vi "peaks.vi"(8 "error in":errorcluster, 9 "List Parameter Fit in":dbl[][](array[numeric]), 10 "List ROI in":dbl[][](array[numeric]), 11 "Spectrum In":cluster{"Locations":dbl[], "Amplitudes":dbl[]}[](array[cluster])=[{"Locations"=array[8192 elements], "Amplitudes"=array[8192 elements]}, {"Locations"=[0.7467606671708176, 1.9235641208245904, 2.29844815204634, 2.952058877083534, 3.30159027268929, 3.693510427204611, 4.0114062030881295, 5.465964569482503, 5.90533601872882, 6.405158056693529, 7.048430896937822, 7.965886489214608, 8.618241797175692, 9.551852093117594, 10.52313535167255, 11.040953037461485, 11.06991514504198, 11.223209663036432, 12.573413841890297, 13.028543500140618, 13.063940211907648, 13.079189646232502, 13.092703597511122, 13.151136366155567, 13.270484104491407, 13.336875706360313, 14.056987568841034, 14.657535881569391, 15.704563469510273, 16.589800479761752, 17.294355204547227, 18.547875406033366, 19.386017685106246, 23.796403305697343, 24.246601838900926, 24.938407230371723], "Amplitudes"=[8249.877716133802, 11327.172305519029, 56622.259938185096, 7573.210585087449, 5296.252862567521, 568942.2217447343, 85362.57126615923, 5991.635098339018, 7019.466820603001, 22054.8389595985, 7981.806397770608, 3443.0618845857953, 7232.474442522111, 1041.175508376075, 20253.913652049327, 2798.643385245958, 2822.1764574507447, 2760.065665975324, 27847.958569595598, 7072.034132274657, 7057.281156133169, 7080.033735934979, 7084.174530276932, 7080.4596184742295, 7256.269557996548, 7151.769553474873, 10957.376602343933, 8796.257531749367, 4885.946335626738, 151185.40382805822, 73397.38735258923, 16617.278737895518, 11305.024780412065, 1494.0162050533122, 1876.7337579234295, 12601.308465489856]}]) -> (0 "error out":errorcluster, 1 "List ROI out":dbl[][](array[numeric]), 2 "Table":string[][](table), 3 "Peaks Out":cluster{"Locations":dbl[], "Amplitudes":dbl[]}, 4 "List Parameter Fit Out":dbl[][](array[numeric]), 6 "Spectrum Fitted":cluster{"Array":dbl[], "Array":dbl[]})   [LabVIEW 2023]
uses:
  <vilib>/Utility/miscctls.llb/LVCursorListTypeDef.ctl
  <vilib>/Utility/miscctls.llb/LVPoint32TypeDef.ctl
  control/global name path.vi
  <vilib>/Utility/cursorutil.llb/Set Cursor (Icon Pict).vi
  <vilib>/Utility/file.llb/Write Delimited Spreadsheet (DBL).vi
  <vilib>/Utility/file.llb/Write Delimited Spreadsheet (string).vi
  <vilib>/Utility/file.llb/Read Delimited Spreadsheet (string).vi
  <vilib>/Utility/file.llb/Read Delimited Spreadsheet (DBL).vi
  queue/Front Panel Message Queue.lvlib
panel:
  out "ROIs":string[][](table)
  out "reference fit panel":refnum<vi>
  in  "previous cursor ID":refnum<k1>
  in  "open":bool
  in  "save":bool
  in  "reset":bool
  out "cluster roi":T1
  in  "mapping":enum16{"Y -Linear", "Y - Log"}(ring)
  in  "eval":bool
  out "grabbing":bool
  in  "Delete":bool
  in  "Normal":bool
  in  "fit":bool
  out "removing":bool
  in  "Stop":bool
  out "Spectrum":cluster{"Locations":dbl[], "Amplitudes":dbl[]}[](graph)
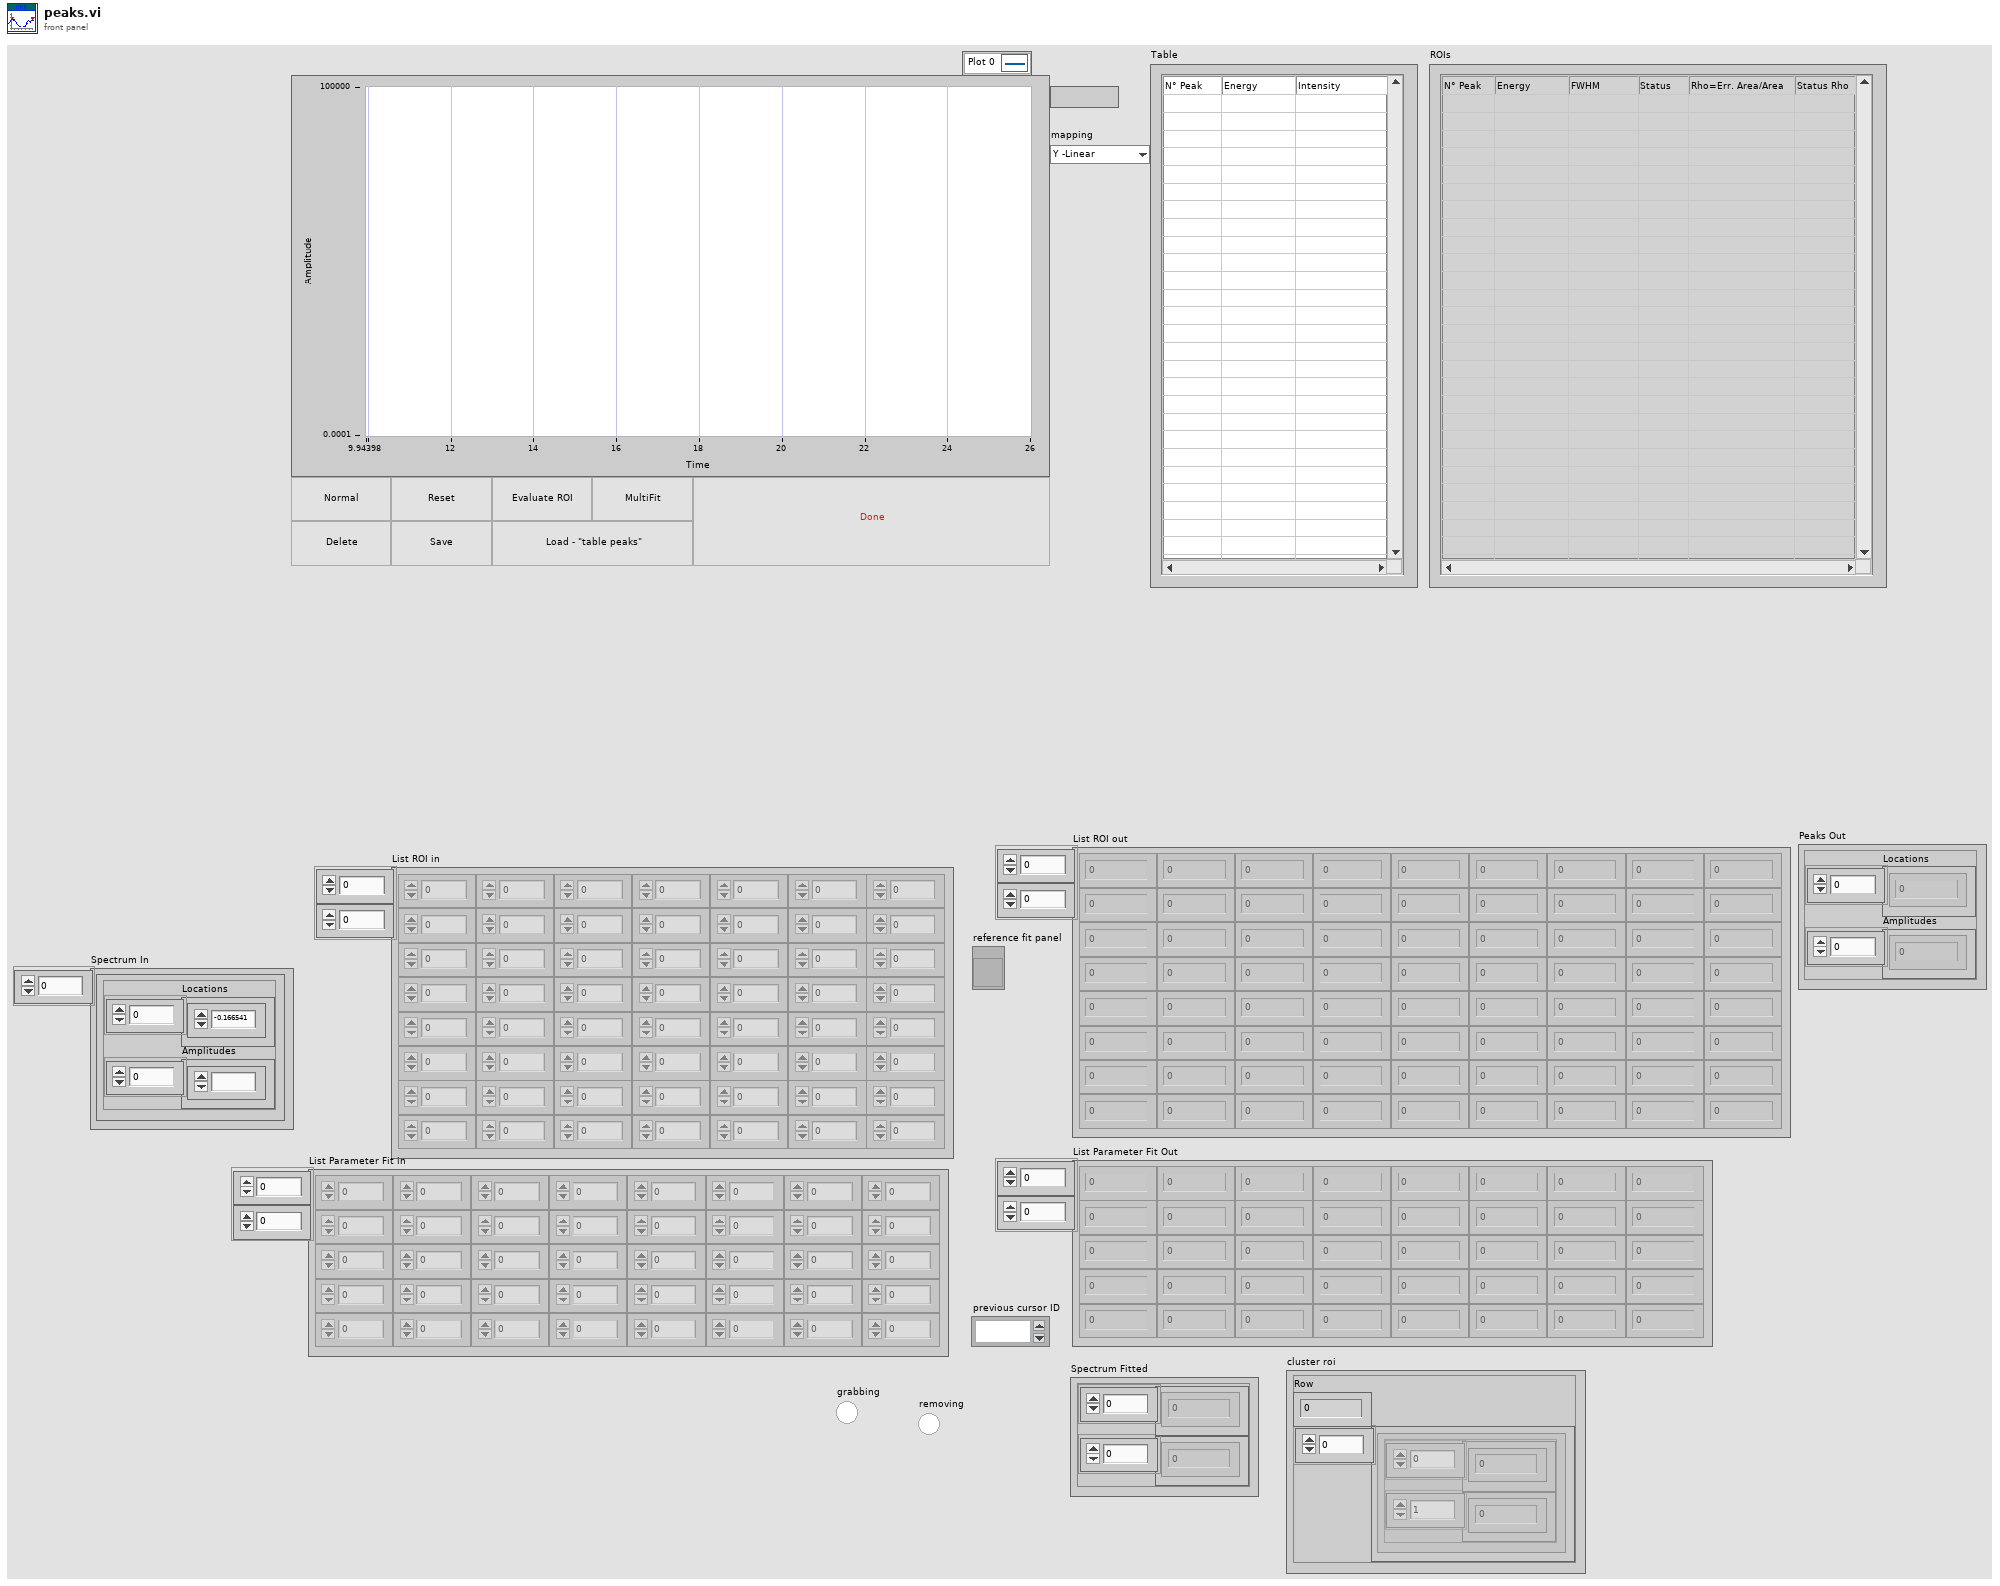
[diagram p1: front panel]
types:
  T1 = cluster{"Row":i32, "Array":cluster{"Array":dbl[], "Array":dbl[]}[]}
  T2 = typedef "Front Panel Message Queue.lvlib/load Message Queues.ctl" = cluster{"Main":refnum<queue>}
  T3 = enum32{"Invalid", "Standard", "Closed", "Hidden", "Minimized", "Maximized"}
  T4 = cluster{"Name":string, "Color":u32, "Style":i32, "Point Style":i32, "Name Visible":bool, "Allow Drag":bool, "Cursor Mode":u32, "Plot":i32, "Index":i32, "Position":cluster{"X":dbl, "Y":dbl}, "X Scale":u32, "Y Scale":u32, "Watch Plots":i32[], "Watch All Plots":bool, "Plot Area":i32, "Label Offset":cluster{"X":dbl, "Y":dbl}}
  T5 = typedef "LVCursorListTypeDef.ctl" = cluster{"Name":string, "Color":u32, "Style":u8, "Point Style":u8, "Name Visible":bool, "Allow Drag":bool, "Cursor Mode":u32, "Plot":i32, "Index":i32, "Position":cluster{"X":dbl, "Y":dbl}, "X Scale":u32, "Y Scale":u32, "Watch Plots":i32[], "Watch All Plots":bool, "Plot Area":i32, "Label Offset":cluster{"X":dbl, "Y":dbl}}[]
  T6 = typedef "LVPoint32TypeDef.ctl" = cluster{"Horizontal":i32, "Vertical":i32}
  T7 = cluster{"Name":string, "Color":u32, "Style":i32, "Point Style":i32, "Name Visible":bool, "Allow Drag":bool, "Cursor Mode":u32, "Plot":i32, "Index":i32, "Position":cluster{"X":dbl, "Y":dbl}, "X Scale":u32, "Y Scale":u32, "Watch Plots":i32[], "Watch All Plots":bool, "Plot Area":i32, "Label Offset":cluster{"X":dbl, "Y":dbl}}[]
  T8 = typedef "LVRowAndColumnTypeDef.ctl" = cluster{"Row":i32, "Column":i32}
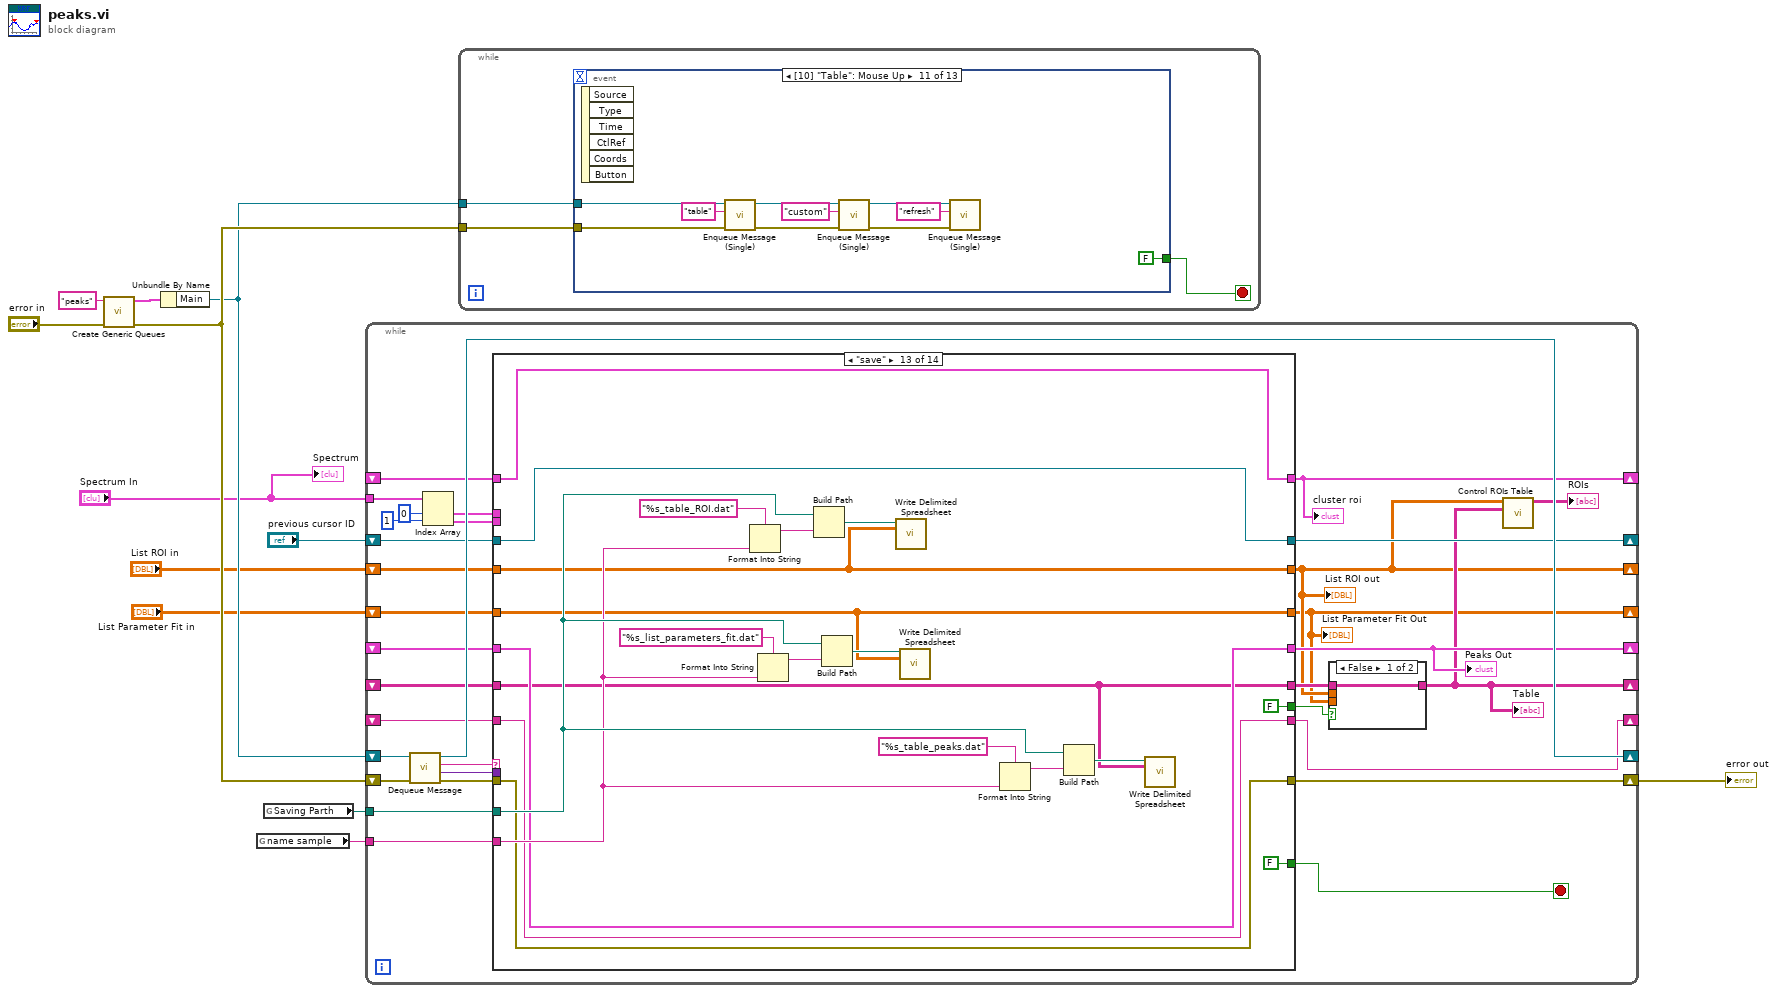
[diagram p0: block diagram]
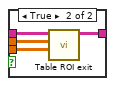
[diagram p2: hidden frame]
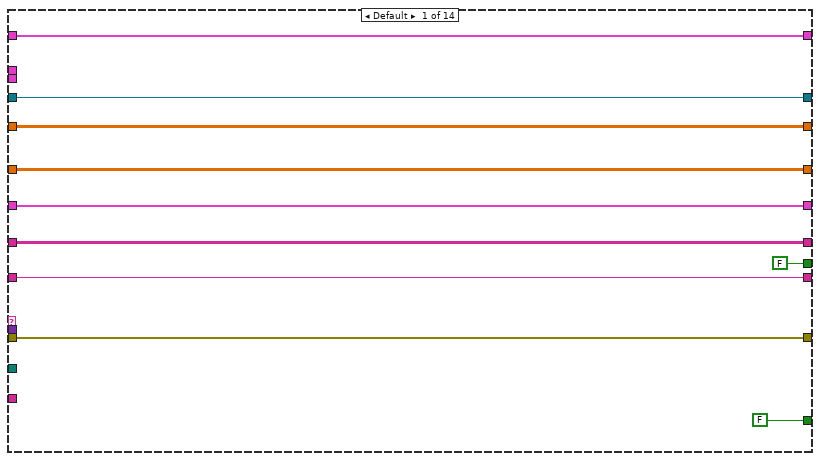
[diagram p3: hidden frame]
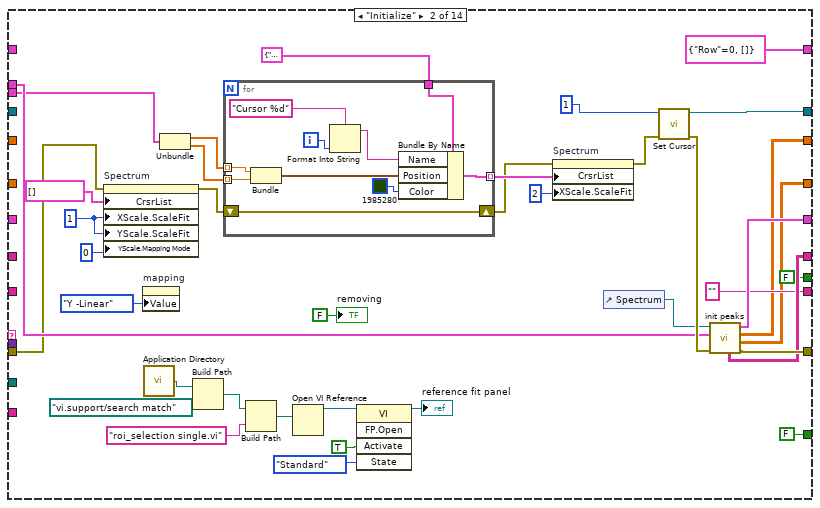
[diagram p4: hidden frame]
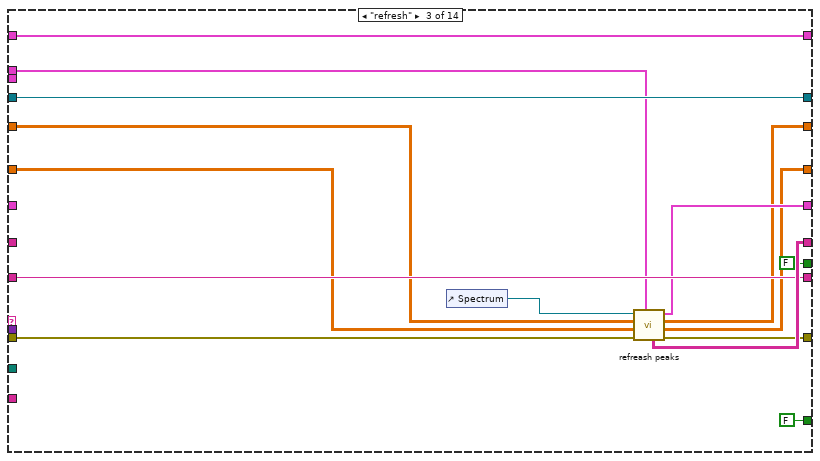
[diagram p5: hidden frame]
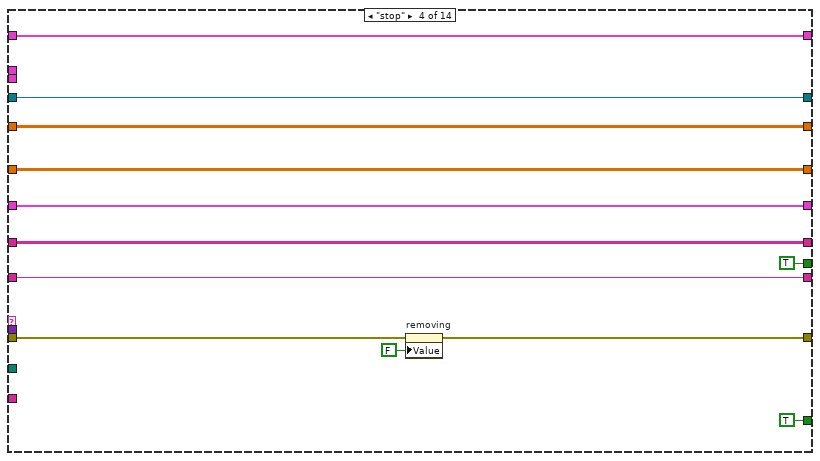
[diagram p6: hidden frame]
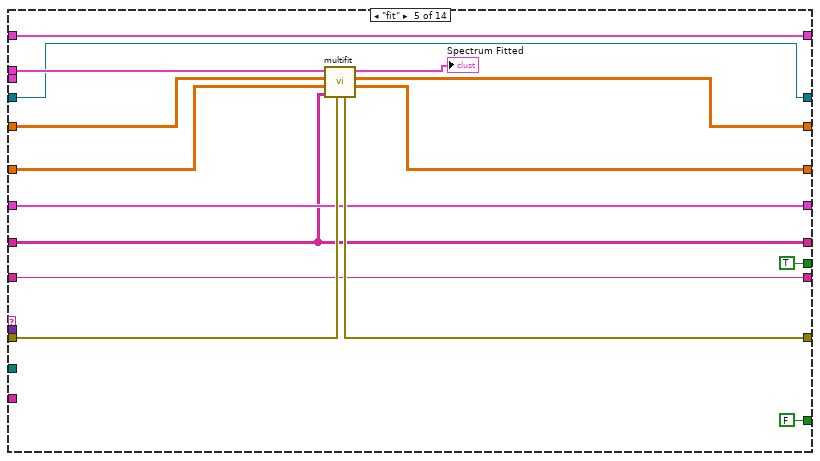
[diagram p7: hidden frame]
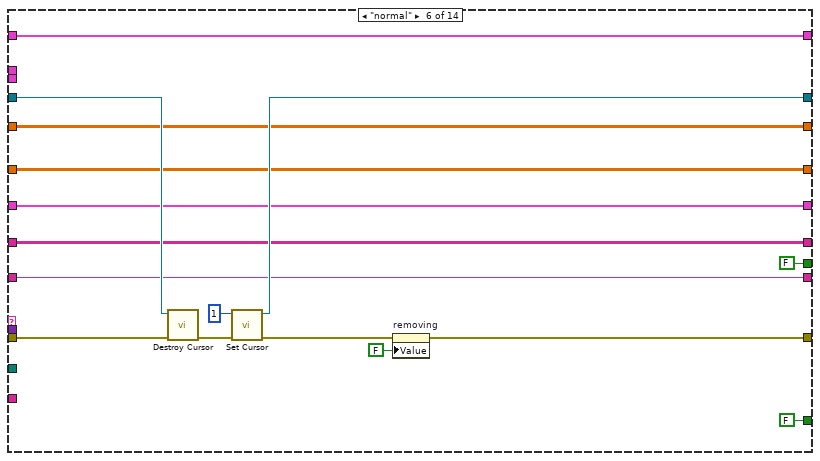
[diagram p8: hidden frame]
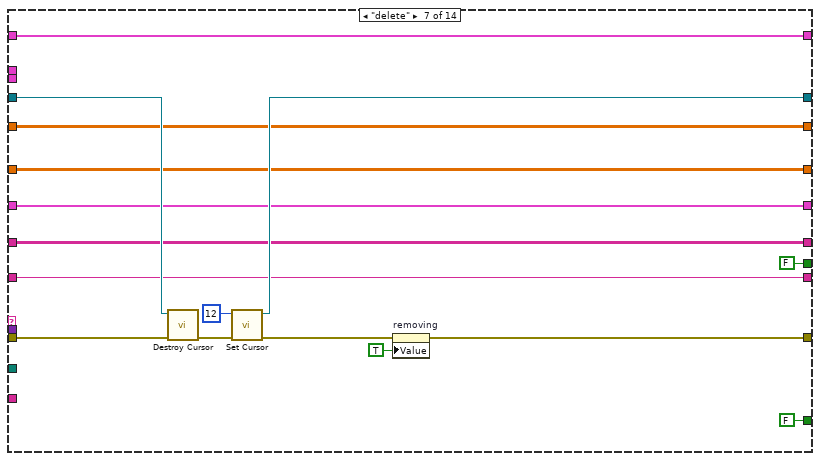
[diagram p9: hidden frame]
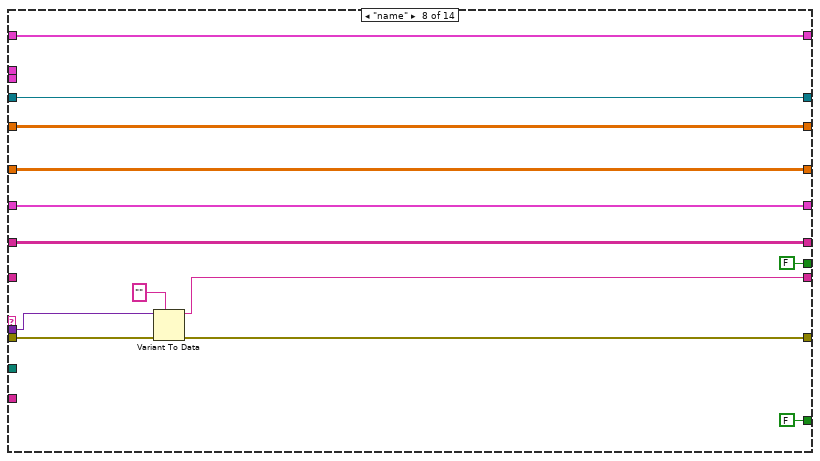
[diagram p10: hidden frame]
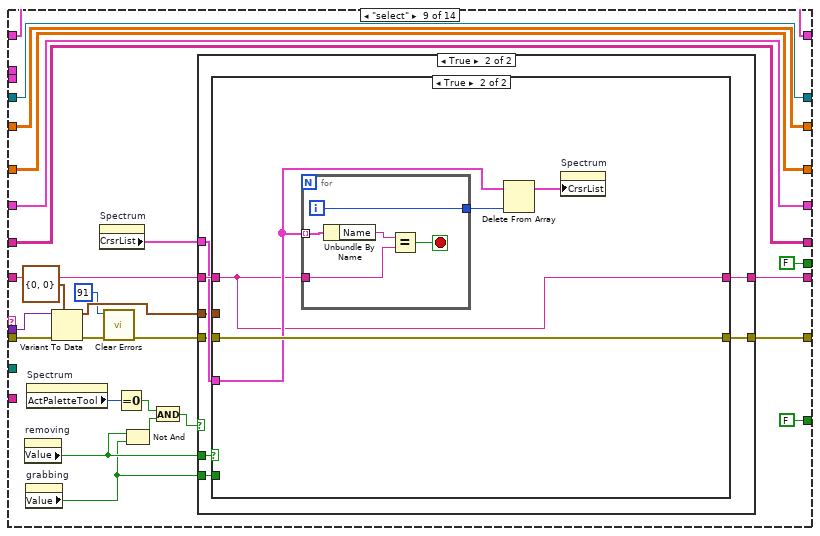
[diagram p11: hidden frame]
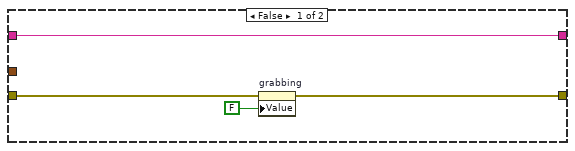
[diagram p12: hidden frame]
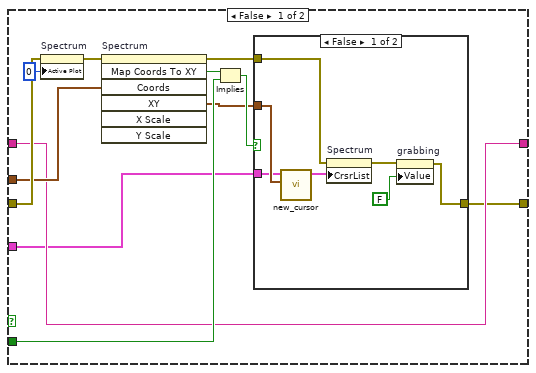
[diagram p13: hidden frame]
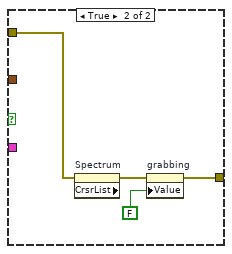
[diagram p14: hidden frame]
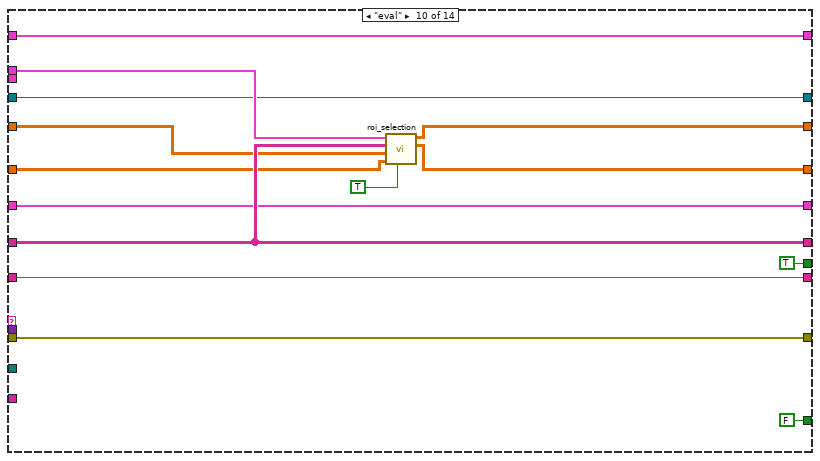
[diagram p15: hidden frame]
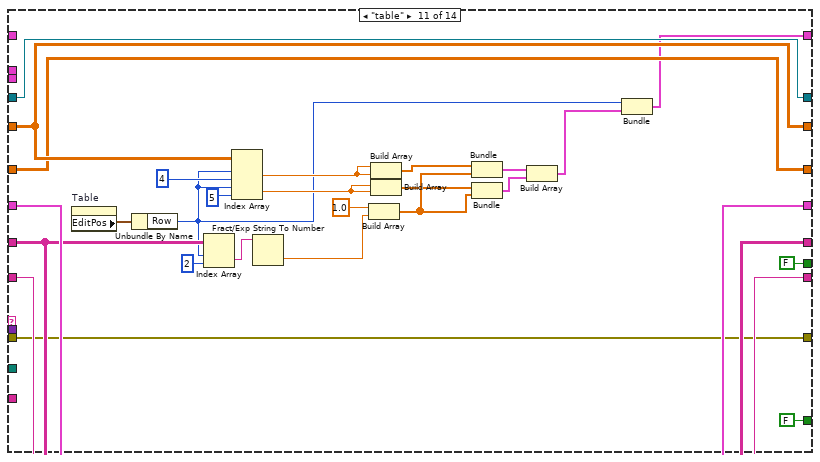
[diagram p16: hidden frame]
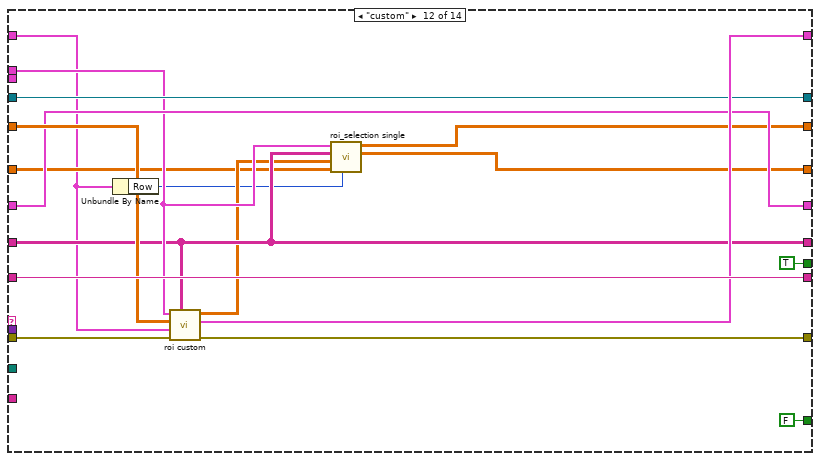
[diagram p17: hidden frame]
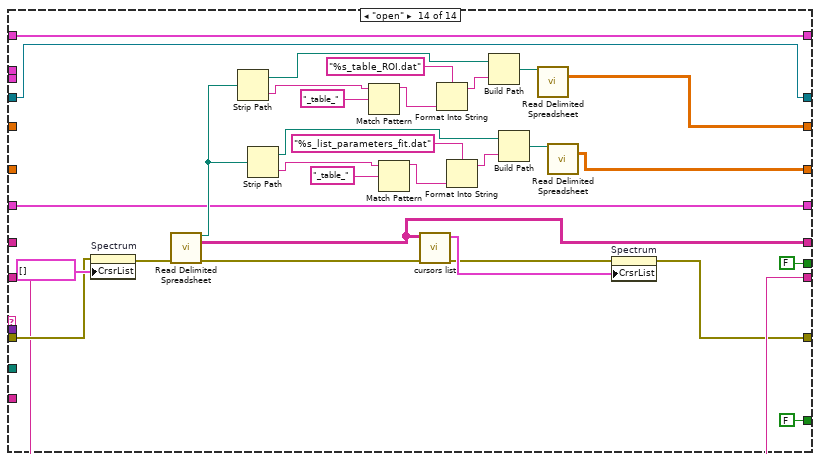
[diagram p18: hidden frame]
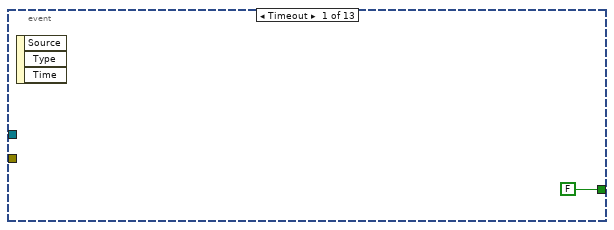
[diagram p19: hidden frame]
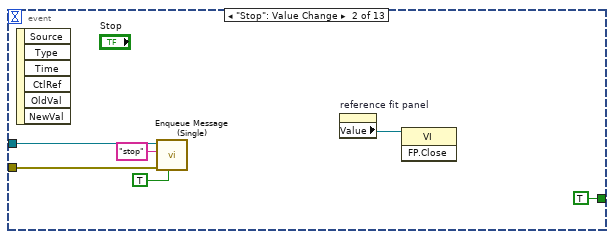
[diagram p20: hidden frame]
diagram:
  n1 = call "Create Generic Queues.vi"("error in (no error)"="error in", "name"="peaks") -> ("error out"=w10:errorcluster, "Message Queues"=w9:T2)  [unwired: 8 in]
  n2 = Unbundle By Name(w9) -> ("Main"=w8:refnum<queue>)
  n3 = global read "global name path.vi" "name sample"() -> (w4:string)
  n4 = global read "global name path.vi" "Saving Parth"() -> (w5:path)
  n5 = while {
    shift-right: [w42] -> _
    shift-left: w8 -> [w43]
    shift-right: [w39] -> w6
    shift-left: w10 -> [w44]
    tunnel: "Spectrum In" -> [w28]
    tunnel: w5 -> [w35]
    tunnel: w4 -> [w36]
    shift-right: [w34] -> _
    shift-left: "previous cursor ID" -> [w33]
    shift-right: [w16] -> _
    shift-left: "List ROI in" -> [w30]
    shift-right: [w15] -> _
    shift-left: "List Parameter Fit in" -> [w29]
    shift-right: [w20] -> _
    shift-left: _ -> [w32]
    shift-right: [w18] -> _
    shift-left: _ -> [w31]
    shift-right: [w14] -> _
    shift-left: _ -> [w23]
    shift-right: [w21] -> _
    shift-left: _ -> [w22]
    stop <- w38 stop-if-true
    n6 = call "Dequeue Message.vi"("error in (no error)"=w44, "Message Queue"=w43) -> ("error out"=w40:errorcluster, "Message Data"=w37:variant, "Message"=w41:string, "dup Message Queue"=w42:refnum<queue>)  [unwired: 5 in, 1 out]
    n7 = Index Array(array=w28, index #1=0 ("index"), index #2=1 ("index")) -> (element #1=w25:cluster{"Locations":dbl[], "Amplitudes":dbl[]}, element #2=w24:cluster{"Locations":dbl[], "Amplitudes":dbl[]})
    n8 = case shown="\"save\"" w41 {
      tunnel: w40 -> [w59 w75 w119 w129 w145 w162 w178 w193 w218 w272 w285 w320 w330 w371]
      tunnel: [w59 w85 w113 w130 w144 w154 w170 w189 w215 w272 w285 w319 w330 w344] -> w39
      tunnel: [FALSE FALSE FALSE TRUE FALSE FALSE FALSE FALSE FALSE FALSE FALSE FALSE FALSE FALSE] -> w38
      tunnel: w37 -> [_ _ _ _ _ _ _ w192 w217 _ _ _ _ _]
      tunnel: w36 -> [_ _ _ _ _ _ _ _ _ _ _ _ w332 _]
      tunnel: w35 -> [_ _ _ _ _ _ _ _ _ _ _ _ w333 _]
      tunnel: [w57 w86 w121 w133 w147 w160 w176 w184 w212 w268 w301 w314 w326 w349] -> w34
      tunnel: w33 -> [w57 _ w121 w133 w147 w161 w177 w184 w212 w268 w301 w314 w326 w349]
      tunnel: [w56 w74 w115 w125 w137 w159 w175 w185 w211 w269 w294 w306 w324 w353] -> w16
      tunnel: [w55 w73 w114 w124 w138 w158 w174 w186 w210 w270 w293 w307 w323 w352] -> w15
      tunnel: [w54 w82 w116 w132 w142 w157 w173 w187 w209 w267 w302 w315 w328 w351] -> w20
      tunnel: w32 -> [w54 _ _ w132 w142 w157 w173 w187 w209 w267 w302 w315 w328 w351]
      tunnel: [w53 w81 w118 w126 w136 w156 w172 w188 w208 w276 w297 w312 w325 w347] -> w17
      tunnel: w31 -> [w53 _ _ w126 w136 w156 w172 w188 w208 w276 w297 w312 w325 _]
      tunnel: w30 -> [w56 _ w110 w125 w148 w159 w175 w185 w211 w275 w294 w317 w324 _]
      tunnel: w29 -> [w55 _ w109 w124 w143 w158 w174 w186 w210 w274 w293 w310 w323 _]
      tunnel: w25 -> [_ w79 w111 _ w149 _ _ _ _ w277 _ w313 _ _]
      tunnel: w24 -> [_ w78 _ _ _ _ _ _ _ _ _ _ _ _]
      tunnel: [w52 "" w117 w128 w140 w152 w168 w190 w206 w271 w303 w318 w329 w370] -> w14
      tunnel: w23 -> [w52 _ w117 w128 w140 w152 w168 _ w207 w271 w303 w318 w329 w370]
      tunnel: [w51 cluster{"Row":i32, cluster{dbl[], dbl[]}[]} {"Row"=0, []} w112 w127 w139 w151 w167 w183 w205 w266 w280 w316 w327 w350] -> w21
      tunnel: w22 -> [w51 _ w112 w127 w139 w151 w167 w183 w205 w266 _ w309 w327 w350]
      tunnel: [FALSE FALSE FALSE TRUE TRUE FALSE FALSE FALSE FALSE TRUE FALSE TRUE FALSE FALSE] -> w13
      frame Default {
      }
      frame "Initialize" {
        w96 = u8 1 ("X Scale.Scale Fit")
        n9 = property on="Spectrum" class="XYGraph (strict)"(error in=w75, "CrsrList"=T5 [] ("Cursor List"), "XScale.ScaleFit"=w96, "YScale.ScaleFit"=w96, "YScale.Mapping Mode"=u8 0 ("Y Scale.Mapping Mode")) -> (error out=w91:errorcluster)  [unwired: 1 in, 1 out]
        n10 = property on="mapping" class="Enum (strict)"("Value"=enum16{"Y -Linear", "Y - Log"}."Y -Linear" ("mapping")) -> ()  [unwired: 2 in, 2 out]
        n11 = call <vilib>:"Application Directory.vi"() -> ("Application Directory"=w70:path)
        n12 = Unbundle(w78) -> ("Locations"=w93:dbl[], "Amplitudes"=w92:dbl[])
        n13 = Build Path(base path=w70, name or relative path=path "vi.support/search match") -> (appended path=w67:path)
        n14 = for {
          tunnel: w93 -> [w105] mode=indexing
          tunnel: w92 -> [w104] mode=indexing
          tunnel: T4 {"Name"="", "Color"=16776704, "Style"=4, "Point Style"=13, "Name Visible"=FALSE, "Allow Drag"=TRUE, "Cursor Mode"=0, "Plot"=0, "Index"=0, "Position"={"X"=0.0, "Y"=0.0}, "X Scale"=0, "Y Scale"=0, "Watch Plots"=[], "Watch All Plots"=FALSE, "Plot Area"=0, "Label Offset"={"X"=0.0, "Y"=0.0}} -> [w103]
          tunnel: [w99] -> w90 mode=indexing
          shift-right: [w98] -> w89
          shift-left: w91 -> [w98]
          i -> [w106]
          n15 = Bundle("Numeric Control"=w105, "Numeric"=w104) -> (w100:cluster{"Numeric Control":dbl, "Numeric":dbl})  [unwired: 1 in]
          n16 = Format Into String(format string="Cursor %d", w106) -> (resulting string=w102:string)  [unwired: 2 in, 1 out]
          n17 = Bundle By Name(cluster=w103, "Name"=w102, "Position"=w100, "Color"=u32 1985280) -> (w99:T4)
        }
        n18 = Build Path(base path=w67, name or relative path="roi_selection single.vi") -> (appended path=w66:path)
        n19 = Open VI Reference(vi path=w66) -> (vi reference=w65:refnum<vi>)  [unwired: 5 in, 1 out]
        n20 = invoke class="VI" method="FP.Open"(reference=w65, "Activate"=TRUE ("Activate?"), "State"=T3."Standard") -> (reference out=→"reference fit panel":refnum<vi>)  [unwired: 2 in, 4 out]
        n21 = property on="Spectrum" class="XYGraph (strict)"(error in=w89, "CrsrList"=w90, "XScale.ScaleFit"=u8 2 ("X Scale.Scale Fit")) -> (error out=w88:errorcluster)  [unwired: 1 in, 1 out]
        n22 = control-ref of="Spectrum"() -> (w83:refnum<vi>)
        n23 = call-poly <vilib>:"Set Cursor.vi"("error in (no error)"=w88, "icon"=u16 1) -> ("error out"=w84:errorcluster, "previous cursor ID"=w86:refnum<k1>)  [unwired: 8 in]
        n24 = call "init peaks.vi"("error in"=w84, "element"=w79, "Spectrum"=w83) -> ("error out"=w85:errorcluster, "List Parameter Fit Out"=w73:dbl[][], "List ROI Out"=w74:dbl[][], "Peaks Out"=w82:cluster{"Locations":dbl[], "Amplitudes":dbl[]}, "Table"=w81:string[][])  [unwired: 4 in]
        "removing" <- FALSE ("removing")
      }
      frame "refresh" {
        n25 = control-ref of="Spectrum"() -> (w120:refnum<vi>)
        n26 = call "refreash peaks.vi"("element"=w111, "error in"=w119, "List Parameter Fit in"=w109, "List ROI in"=w110, "Spectrum"=w120) -> ("error out"=w113:errorcluster, "List Parameter Fit Out"=w114:dbl[][], "List ROI Out"=w115:dbl[][], "Peaks Out"=w116:cluster{"Locations":dbl[], "Amplitudes":dbl[]}, "Table"=w118:string[][])  [unwired: 2 in]
      }
      frame "stop" {
        n27 = property on="removing" class="Bool (strict)"(error in=w129, "Value"=FALSE ("removing")) -> (error out=w130:errorcluster)  [unwired: 1 in, 1 out]
      }
      frame "fit" {
        n28 = call "multifit.vi"("error in"=w145, "List Peaks"=w136, "List Parameter Fit In"=w143, "List ROI In"=w148, "Spectrum In"=w149) -> ("List Parameter Fit Out"=w138:dbl[][], "List ROI Out"=w137:dbl[][], "Spectrum Fitted"=→"Spectrum Fitted":cluster{"Array":dbl[], "Array":dbl[]}, "error out"=w144:errorcluster)  [unwired: 3 in]
      }
      frame "normal" {
        n29 = call <vilib>:"Destroy Cursor.vi"("cursor ID"=w161, "error in (no error)"=w162) -> ("error out"=w163:errorcluster)  [unwired: 8 in]
        n30 = call-poly <vilib>:"Set Cursor.vi"("error in (no error)"=w163, "icon"=u16 1 ("Cursor Icon")) -> ("error out"=w153:errorcluster, "previous cursor ID"=w160:refnum<k1>)  [unwired: 8 in]
        n31 = property on="removing" class="Bool (strict)"(error in=w153, "Value"=FALSE ("removing")) -> (error out=w154:errorcluster)  [unwired: 1 in, 1 out]
      }
      frame "delete" {
        n32 = call <vilib>:"Destroy Cursor.vi"("cursor ID"=w177, "error in (no error)"=w178) -> ("error out"=w179:errorcluster)  [unwired: 8 in]
        n33 = call-poly <vilib>:"Set Cursor.vi"("error in (no error)"=w179, "icon"=u16 12 ("Cursor Icon")) -> ("error out"=w169:errorcluster, "previous cursor ID"=w176:refnum<k1>)  [unwired: 8 in]
        n34 = property on="removing" class="Bool (strict)"(error in=w169, "Value"=TRUE ("removing")) -> (error out=w170:errorcluster)  [unwired: 1 in, 1 out]
      }
      frame "name" {
        n35 = Variant To Data(error in=w193, type="", Variant=w192) -> (data=w190:string, error out=w189:errorcluster)
      }
      frame "select" {
        n36 = property on="removing" class="Bool (strict)"() -> ("Value"=w200:bool)  [unwired: 2 in, 2 out]
        n37 = property on="grabbing" class="Bool (strict)"() -> ("Value"=w199:bool)  [unwired: 2 in, 2 out]
        n38 = property on="Spectrum" class="XYGraph (strict)"() -> ("ActPaletteTool"=w216:i32)  [unwired: 2 in, 2 out]
        n39 = Variant To Data(error in=w218, type=T6 {"Horizontal"=0, "Vertical"=0} ("Coords"), Variant=w217) -> (data=w214:T6, error out=w203:errorcluster)
        n40 = property on="Spectrum" class="XYGraph (strict)"() -> ("CrsrList"=w213:T5)  [unwired: 2 in, 2 out]
        n41 = call <vilib>:"Clear Errors.vi"("error in (no error)"=w203, "specific error code to clear (0: all)"=91) -> ("error out"=w202:errorcluster)  [unwired: 4 in, 1 out]
        n42 = Equal To 0?(x=w216) -> (x = 0?=w198:bool)
        n43 = Not And(1:w199, 2:w200) -> (0:w197:bool)
        n44 = And(x=w198, y=w197) -> (x .and. y?=w196:bool)
        n45 = case shown="True" w196 {
          tunnel: w202 -> [w221 w227]
          tunnel: [w220 w228] -> w215
          tunnel: w214 -> [_ w225]
          tunnel: w213 -> [_ w229]
          tunnel: w207 -> [w223 w230]
          tunnel: w200 -> [_ w231]
          tunnel: [w223 w226] -> w206
          tunnel: w199 -> [_ w224]
          frame False {
            n46 = property on="grabbing" class="Bool (strict)"(error in=w221, "Value"=FALSE ("grabbing")) -> (error out=w220:errorcluster)  [unwired: 1 in, 1 out]
          }
          frame True {
            n47 = case shown="True" w231 {
              tunnel: w230 -> [w237 w255]
              tunnel: w229 -> [w233 w257]
              tunnel: [w235 w259] -> w228
              tunnel: w227 -> [w242 w259]
              tunnel: [w237 w255] -> w226
              tunnel: w225 -> [w240 _]
              tunnel: w224 -> [w238 _]
              frame False {
                n48 = property on="Spectrum" class="XYGraph (strict)"(error in=w242, "Active Plot"=u32 0) -> (error out=w241:errorcluster)  [unwired: 1 in, 1 out]
                n49 = invoke on="Spectrum" class="XYGraph (strict)" method="Map Coords To XY"(error in=w241, "Coords"=w240) -> (error out=w234:errorcluster, "Map Coords To XY"=w239:bool, "XY"=w232:cluster{"X":dbl, "Y":dbl})  [unwired: 5 in, 4 out]
                n50 = Implies(1:w238, 2:w239) -> (0:w236:bool)
                n51 = case shown="False" w236 {
                  tunnel: [w244 w251] -> w235
                  tunnel: w234 -> [w247 w254]
                  tunnel: w233 -> [w249 _]
                  tunnel: w232 -> [w250 _]
                  frame False {
                    n52 = call "new_cursor.vi"("XY"=w250, "CrsrList"=w249) -> ("CrsrList Out"=w248:T7)  [unwired: 9 in]
                    n53 = property on="Spectrum" class="XYGraph (strict)"(error in=w247, "CrsrList"=w248) -> (error out=w246:errorcluster)  [unwired: 1 in, 1 out]
                    n54 = property on="grabbing" class="Bool (strict)"(error in=w246, "Value"=FALSE ("grabbing")) -> (error out=w244:errorcluster)  [unwired: 1 in, 1 out]
                  }
                  frame True {
                    n55 = property on="Spectrum" class="XYGraph (strict)" props=["CrsrList"](error in=w254) -> (error out=w252:errorcluster)  [unwired: 1 in, 2 out]
                    n56 = property on="grabbing" class="Bool (strict)"(error in=w252, "Value"=FALSE ("grabbing")) -> (error out=w251:errorcluster)  [unwired: 1 in, 1 out]
                  }
                }
              }
              frame True {
                n57 = for {
                  tunnel: w257 -> [w264] mode=indexing
                  tunnel: w255 -> [w262]
                  tunnel: [w260] -> w258
                  i -> [w260]
                  stop <- w261 stop-if-true
                  n58 = Unbundle By Name(w264) -> ("Name"=w263:string)
                  n59 = Equal?(x=w263, y=w262) -> (x = y?=w261:bool)
                }
                n60 = Delete From Array(array=w257, index=w258) -> (array with subset deleted=w256:T5)  [unwired: 1 in, 1 out]
                n61 = property on="Spectrum" class="XYGraph (strict)"("CrsrList"=w256) -> ()  [unwired: 2 in, 2 out]
              }
            }
          }
        }
      }
      frame "eval" {
        n62 = call "roi_selection.vi"("Starting Evaluate?"=TRUE, "List Parameter Fit In"=w274, "List ROI In"=w275, "List Peaks"=w276, "Spectrum In"=w277) -> ("List Parameter Fit Out"=w270:dbl[][], "List ROI Out"=w269:dbl[][])  [unwired: 5 in]
      }
      frame "table" {
        n63 = property on="Table" class="Tbl (strict)"() -> ("EditPos"=w300:T8)  [unwired: 2 in, 2 out]
        n64 = Unbundle By Name(w300) -> ("Row"=w281:i32)
        n65 = Index Array(array=w297, index (row)=w281, index (col)=2 ("disabled index (col)")) -> (element=w299:string)
        n66 = Index Array(array=w294, index (row) #1=w281, index (col) #1=4 ("disabled index (col)"), index (row) #2=w281, index (col) #2=5 ("disabled index (col)")) -> (element #1=w288:dbl, element #2=w287:dbl)
        n67 = Fract/Exp String To Number(string=w299) -> (number=w286:dbl)  [unwired: 3 in, 1 out]
        n68 = Build Array(1.0, w286) -> (w292:dbl[])
        n69 = Build Array(w288, w288) -> (w289:dbl[])
        n70 = Build Array(w287, w287) -> (w291:dbl[])
        n71 = Bundle(w289, w292) -> (w284:cluster{dbl[], dbl[]})  [unwired: 1 in]
        n72 = Bundle(w291, w292) -> (w283:cluster{dbl[], dbl[]})  [unwired: 1 in]
        n73 = Build Array(w284, w283) -> (w282:cluster{dbl[], dbl[]}[])
        n74 = Bundle("Row"=w281, w282) -> (w280:cluster{"Row":i32, cluster{dbl[], dbl[]}[]})  [unwired: 1 in]
      }
      frame "custom" {
        n75 = Unbundle By Name(w309) -> ("Row"=w308:i32)
        n76 = call "roi custom.vi"("Table"=w312, "Error In"=w320, "Cluster roi in"=w309, "List ROI In"=w317, "Spectrum In"=w313) -> ("Error Out"=w319:errorcluster, "Cluster roi out"=w316:T1, "List ROI Out"=w311:dbl[][])  [unwired: 4 in]
        n77 = call "roi_selection single.vi"("Peak selected"=w308, "List Parameter Fit In"=w310, "List ROI In"=w311, "List Peaks"=w312, "Spectrum In"=w313) -> ("List Parameter Fit Out"=w307:dbl[][], "List ROI Out"=w306:dbl[][])  [unwired: 5 in]
      }
      frame "save" {
        n78 = Format Into String(format string="%s_table_ROI.dat", w332) -> (resulting string=w342:string)  [unwired: 2 in, 1 out]
        n79 = Format Into String(format string="%s_list_parameters_fit.dat", w332) -> (resulting string=w336:string)  [unwired: 2 in, 1 out]
        n80 = Build Path(base path=w333, name or relative path=w342) -> (appended path=w340:path)
        n81 = Build Path(base path=w333, name or relative path=w336) -> (appended path=w334:path)
        n82 = call-poly <vilib>:"Write Delimited Spreadsheet.vi"("file path (dialog if empty)"=w340, "2D data"=w324) -> ()  [unwired: 12 in, 2 out]
        n83 = call-poly <vilib>:"Write Delimited Spreadsheet.vi"("file path (dialog if empty)"=w334, "2D data"=w323) -> ()  [unwired: 12 in, 2 out]
        n84 = Format Into String(format string="%s_table_peaks.dat", w332) -> (resulting string=w337:string)  [unwired: 2 in, 1 out]
        n85 = Build Path(base path=w333, name or relative path=w337) -> (appended path=w339:path)
        n86 = call-poly <vilib>:"Write Delimited Spreadsheet.vi"("file path (dialog if empty)"=w339, "2D data"=w325) -> ()  [unwired: 12 in, 2 out]
      }
      frame "open" {
        n87 = property on="Spectrum" class="XYGraph (strict)"(error in=w371, "CrsrList"=T5 [] ("Cursor List")) -> (error out=w372:errorcluster)  [unwired: 1 in, 1 out]
        n88 = call-poly <vilib>:"Read Delimited Spreadsheet.vi"("error in (no error)"=w372) -> ("new file path (Not A Path if cancelled)"=w354:path, "all rows"=w347:string[][], "error out"=w348:errorcluster)  [unwired: 9 in, 3 out]
        n89 = Strip Path(path=w354) -> (stripped path=w367:path, name=w365:string)
        n90 = Strip Path(path=w354) -> (stripped path=w356:path, name=w358:string)
        n91 = Match Pattern(string=w365, regular expression="_table_" ("format string")) -> (before substring=w364:string)  [unwired: 1 in, 3 out]
        n92 = Match Pattern(string=w358, regular expression="_table_" ("format string")) -> (before substring=w359:string)  [unwired: 1 in, 3 out]
        n93 = call "cursors list.vi"("error in"=w348, "Table"=w347) -> ("error out"=w345:errorcluster, "Cursors List"=w346:T7)  [unwired: 8 in]
        n94 = Format Into String(format string="%s_table_ROI.dat", w364) -> (resulting string=w366:string)  [unwired: 2 in, 1 out]
        n95 = Format Into String(format string="%s_list_parameters_fit.dat", w359) -> (resulting string=w357:string)  [unwired: 2 in, 1 out]
        n96 = Build Path(base path=w367, name or relative path=w366) -> (appended path=w368:path)
        n97 = Build Path(base path=w356, name or relative path=w357) -> (appended path=w355:path)
        n98 = call-poly <vilib>:"Read Delimited Spreadsheet.vi"("file path (dialog if empty)"=w368) -> ("all rows"=w353:dbl[][])  [unwired: 9 in, 5 out]
        n99 = call-poly <vilib>:"Read Delimited Spreadsheet.vi"("file path (dialog if empty)"=w355) -> ("all rows"=w352:dbl[][])  [unwired: 9 in, 5 out]
        n100 = property on="Spectrum" class="XYGraph (strict)"(error in=w345, "CrsrList"=w346) -> (error out=w344:errorcluster)  [unwired: 1 in, 1 out]
      }
    }
    "cluster roi" <- w21
    "Peaks Out" <- w20
    "List Parameter Fit Out" <- w15
    "List ROI out" <- w16
    n101 = case shown="False" w13 {
      tunnel: [w45 w49] -> w18
      tunnel: w17 -> [w45 w48]
      tunnel: w16 -> [_ w47]
      tunnel: w15 -> [_ w46]
      frame False {
      }
      frame True {
        n102 = call "Table ROI exit.vi"("List Parameter Fit In"=w46, "List ROI In"=w47, "Table In"=w48) -> ("Table Out"=w49:string[][])  [unwired: 8 in]
      }
    }
    "Table" <- w18
    n103 = call "Control ROIs Table.vi"("Table"=w18, "List ROI in"=w16) -> ("ROIs"=→"ROIs":string[][])  [unwired: 9 in]
  }
  "error out" <- w6
  n104 = while {
    tunnel: w10 -> [w375]
    tunnel: w8 -> [w374]
    stop <- w376 stop-if-true
    n105 = event shown="[10] \"Table\": Mouse Up" {
      selector: _ -> [_ _ _ _ _ _ _ _ _ _ _ _ _]
      dyn-events: _ -> [_ _ _ _ _ _ _ _ _ _ _ _ _]
      timeout: _ -> [_ _ _ _ _ _ _ _ _ _ _ _ _]
      tunnel: [FALSE TRUE FALSE FALSE FALSE FALSE FALSE FALSE FALSE FALSE FALSE FALSE FALSE] -> w376
      tunnel: w375 -> [_ w382 w386 w391 w393 w397 w411 w421 w428 _ w441 w445 w449]
      tunnel: w374 -> [_ w383 w385 w390 w394 w398 w410 w420 w429 _ w440 w446 w450]
      event Timeout {
        n106 = event-data() -> ()  [unwired: 1 in, 3 out]
      }
      event "Stop": Value Change {
        n107 = event-data() -> ()  [unwired: 1 in, 6 out]
        n108 = call "Enqueue Message (Single).vi"("Priority Message? (F)"=TRUE, "error in (no error)"=w382, "Message"="stop", "Message Queue"=w383) -> ()  [unwired: 6 in, 2 out]
        n109 = property on="reference fit panel" class="VIRef (strict)"() -> ("Value"=w378:refnum<vi>)  [unwired: 2 in, 2 out]
        n110 = invoke class="VI" method="FP.Close"(reference=w378) -> ()  [unwired: 2 in, 3 out]
      }
      event "reset": Value Change {
        n111 = event-data() -> ()  [unwired: 1 in, 6 out]
        n112 = call "Enqueue Message (Single).vi"("error in (no error)"=w386, "Message"="initialize", "Message Queue"=w385) -> ()  [unwired: 7 in, 2 out]
      }
      event "fit": Value Change {
        n113 = event-data() -> ()  [unwired: 1 in, 6 out]
        n114 = call "Enqueue Message (Single).vi"("error in (no error)"=w391, "Message"="fit", "Message Queue"=w390) -> ()  [unwired: 7 in, 2 out]
      }
      event "Normal": Value Change {
        n115 = event-data() -> ()  [unwired: 1 in, 6 out]
        n116 = call "Enqueue Message (Single).vi"("error in (no error)"=w393, "Message"="normal", "Message Queue"=w394) -> ()  [unwired: 7 in, 2 out]
      }
      event "Delete": Value Change {
        n117 = event-data() -> ()  [unwired: 1 in, 6 out]
        n118 = call "Enqueue Message (Single).vi"("error in (no error)"=w397, "Message"="delete", "Message Queue"=w398) -> ()  [unwired: 7 in, 2 out]
      }
      event "Spectrum": event type 3.0.x80000027 {
        n119 = event-data() -> ("CursRef"=w412:refnum<vi>)  [unwired: 1 in, 3 out]
        n120 = property class="Curs"(reference=w412) -> ("Cursor Name"=w408:string)  [unwired: 1 in, 2 out]
        n121 = To Variant(anything=w408) -> (Variant=w407:variant)
        n122 = call "Enqueue Message (Single).vi"("error in (no error)"=w411, "Message Data"=w407, "Message"="name", "Message Queue"=w410) -> ("error out"=w405:errorcluster, "dup Message Queue"=w404:refnum<queue>)  [unwired: 6 in]
        n123 = call "Enqueue Message (Single).vi"("error in (no error)"=w405, "Message"="select", "Message Queue"=w404) -> ("error out"=w402:errorcluster, "dup Message Queue"=w401:refnum<queue>)  [unwired: 7 in]
        n124 = call "Enqueue Message (Single).vi"("error in (no error)"=w402, "Message"="refresh", "Message Queue"=w401) -> ()  [unwired: 7 in, 2 out]
        n125 = event-data() -> ()  [unwired: 2 in, 1 out]
        "grabbing" <- TRUE ("grabbing")
      }
      event "Spectrum": Mouse Up {
        n126 = event-data() -> ("Coords"=w418:T6)  [unwired: 1 in]
        n127 = To Variant(anything=w418) -> (Variant=w417:variant)
        n128 = call "Enqueue Message (Single).vi"("error in (no error)"=w421, "Message Data"=w417, "Message"="select", "Message Queue"=w420) -> ("error out"=w415:errorcluster, "dup Message Queue"=w414:refnum<queue>)  [unwired: 6 in]
        n129 = call "Enqueue Message (Single).vi"("error in (no error)"=w415, "Message"="refresh", "Message Queue"=w414) -> ()  [unwired: 7 in, 2 out]
      }
      event "eval": Value Change {
        n130 = event-data() -> ()  [unwired: 1 in, 4 out]
        n131 = call "Enqueue Message (Single).vi"("error in (no error)"=w428, "Message"="eval", "Message Queue"=w429) -> ("error out"=w425:errorcluster, "dup Message Queue"=w424:refnum<queue>)  [unwired: 7 in]
        n132 = call "Enqueue Message (Single).vi"("error in (no error)"=w425, "Message"="refresh", "Message Queue"=w424) -> ()  [unwired: 7 in, 2 out]
      }
      event "mapping": Value Change {
        n133 = event-data() -> ("NewVal"=w432:enum16{"Y -Linear", "Y - Log"})  [unwired: 1 in, 5 out]
        n134 = property on="Spectrum" class="XYGraph (strict)"("YScale.Mapping Mode"=w432, "YScale.ScaleFit"=u8 1 ("Y Scale.Scale Fit")) -> ()  [unwired: 2 in, 2 out]
      }
      event "Table": Mouse Up {
        n135 = event-data() -> ()  [unwired: 1 in, 6 out]
        n136 = call "Enqueue Message (Single).vi"("error in (no error)"=w441, "Message"="table", "Message Queue"=w440) -> ("error out"=w438:errorcluster, "dup Message Queue"=w437:refnum<queue>)  [unwired: 7 in]
        n137 = call "Enqueue Message (Single).vi"("error in (no error)"=w438, "Message"="custom", "Message Queue"=w437) -> ("error out"=w436:errorcluster, "dup Message Queue"=w435:refnum<queue>)  [unwired: 7 in]
        n138 = call "Enqueue Message (Single).vi"("error in (no error)"=w436, "Message"="refresh", "Message Queue"=w435) -> ()  [unwired: 7 in, 2 out]
      }
      event "save": Value Change {
        n139 = event-data() -> ()  [unwired: 1 in, 6 out]
        n140 = call "Enqueue Message (Single).vi"("error in (no error)"=w445, "Message"="save", "Message Queue"=w446) -> ()  [unwired: 7 in, 2 out]
      }
      event "open": Value Change {
        n141 = event-data() -> ()  [unwired: 1 in, 6 out]
        n142 = call "Enqueue Message (Single).vi"("error in (no error)"=w449, "Message"="open", "Message Queue"=w450) -> ()  [unwired: 7 in, 2 out]
      }
    }
  }
  "Spectrum" <- "Spectrum In"
